vi "serialization tests.vi"() -> ()   [LabVIEW 2013, in "tag select module tests.lvlib"]
uses:
  tag select module tests.lvlib
  module/configuration/tag select module configuration.lvclass
panel:
  out "size(s) 2":i32
  out "size(s)":i32
  out "modules equal":bool
  out "channels equal":bool
  out "no error":errorcluster
  out "no error":errorcluster
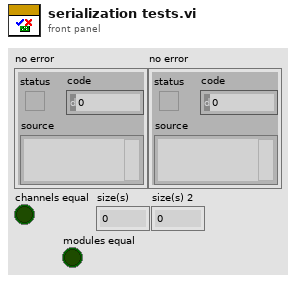
[diagram p1: front panel]
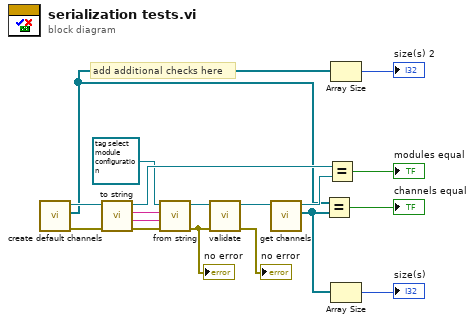
[diagram p0: block diagram]
diagram:
  # "add additional checks here"
  n1 = call "create default channels.vi"() -> ("error out"=w9:errorcluster, "channels"=w4:refnum<class "TBM channel.lvclass">[], "module"=w10:refnum<class "tag select module configuration.lvclass">)  [unwired: 8 in, 1 out]
  n2 = call-dynamic "to string.vi"("error in"=w9, "tag select module configuration in"=w10) -> ("error out"=w18:errorcluster, "data"=w17:string, "version"=w16:string, "tag select module configuration out"=w6:refnum<class "tag select module configuration.lvclass">)  [unwired: 6 in]
  n3 = call-dynamic "from string.vi"("error in"=w18, "data"=w17, "version"=w16, "tag select module configuration in"=refnum<class "tag select module configuration.lvclass"> refnum ("tag bus configurable plugin module configuration")) -> ("error out"=w13:errorcluster, "tag select module configuration out"=w15:refnum<class "tag select module configuration.lvclass">)  [unwired: 6 in]
  "no error" <- w13
  n4 = call-dynamic "validate.vi"("error in"=w13, "alarms module configuration in"=w15) -> ("error out"=→"no error":errorcluster, "alarms module configuration out"=w11:refnum<class "tag select module configuration.lvclass">)  [unwired: 8 in]
  n5 = call-dynamic "get channels.vi"("alarms module configuration in"=w11) -> ("channels"=w3:refnum<class "TBM channel.lvclass">[], "alarms module configuration out"=w7:refnum<class "tag select module configuration.lvclass">)  [unwired: 9 in]
  n6 = Equal?(x=w4, y=w3) -> (x = y?=→"channels equal":bool)
  n7 = Equal?(x=w6, y=w7) -> (x = y?=→"modules equal":bool)
  n8 = Array Size(array=w4) -> (size(s)=→"size(s) 2":i32)
  n9 = Array Size(array=w3) -> (size(s)=→"size(s)":i32)
